vi "resetConjugat.vi"(3 "input":sgl[][](array[numeric]), 4 "ptr":i64, 5 "error in (no error)":errorcluster) -> (0 "input out":sgl[][](array[numeric]), 1 "ptr out":i64, 2 "error out":errorcluster)   [LabVIEW 2016, in "CNet.lvlib"]
uses:
  CNet.lvlib
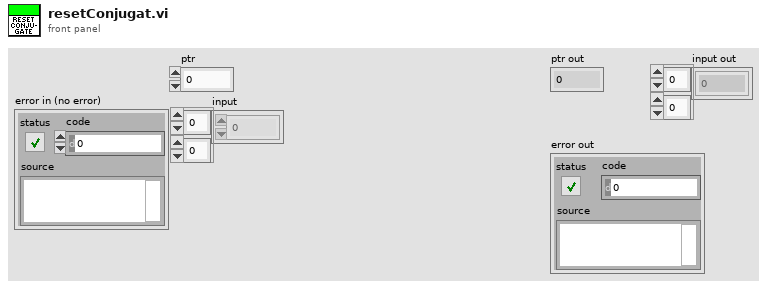
[diagram p1: front panel]
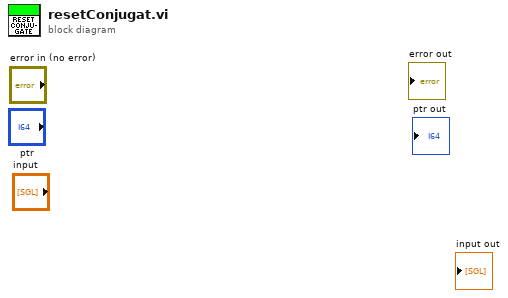
[diagram p0: block diagram]
diagram:
